vi "PH_PSDBWriter.set Thread Command.vi"(3 "error in (no error)":errorcluster, 4 "PSDB Thread Command":T1 items=["None", "GetInstanceID", "WriteToPSDB"], 5 "Queue in":refnum<queue>) -> (0 "error out":errorcluster)   [LabVIEW 2014, in "PH_PSDBWriter.lvlib"]
uses:
  PH_PSDBWriter.lvlib
  PH_PSDBWriter.Thread Commands.ctl
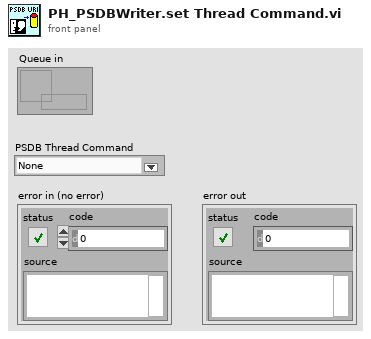
[diagram p1: front panel]
types:
  T1 = typedef "PH_PSDBWriter.lvlib/PH_PSDBWriter.Thread Commands.ctl" = u16
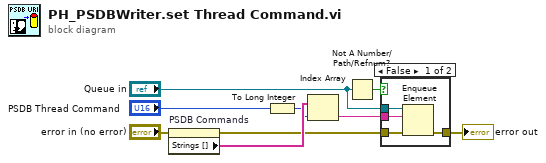
[diagram p0: block diagram]
diagram:
  n1 = property on="PSDB Commands" class="Ring (strict)"(error in="error in (no error)") -> (error out=w2:errorcluster, "Strings []"=w4:string[])  [unwired: 1 in, 1 out]
  n2 = To Long Integer(number="PSDB Thread Command") -> (32bit integer=w1:i32)
  n3 = Index Array(array=w4, index=w1) -> (element=w5:string)
  n4 = Not A Number/Path/Refnum?(number/path/refnum="Queue in") -> (NaN/Path/Refnum?=w9:bool)
  n5 = case shown="False" w9 {
    tunnel: [w13 w14] -> w7
    tunnel: w2 -> [w12 w14]
    tunnel: "Queue in" -> [w11 _]
    tunnel: w5 -> [w10 _]
    frame False {
      n6 = Enqueue Element(queue=w11, element=w10, error in (no error)=w12) -> (error out=w13:errorcluster)  [unwired: 1 in, 2 out]
    }
    frame True {
    }
  }
  "error out" <- w7
